vi "Target Defender Out.vi"(6 "Target Fora in":bool=TRUE, 8 "Field Size in":T1, 9 "Defensores":u32[](array[numeric]), 10 "total":i32, 11 "Ball":dbl[](array[numeric])) -> (2 "Target Fora out":bool=TRUE)   [LabVIEW 2016]
uses:
  Core/Field Size.ctl
panel:
  in  "Campo/2":dbl
  out "Posição dos Defensores":dbl[][](array[numeric])
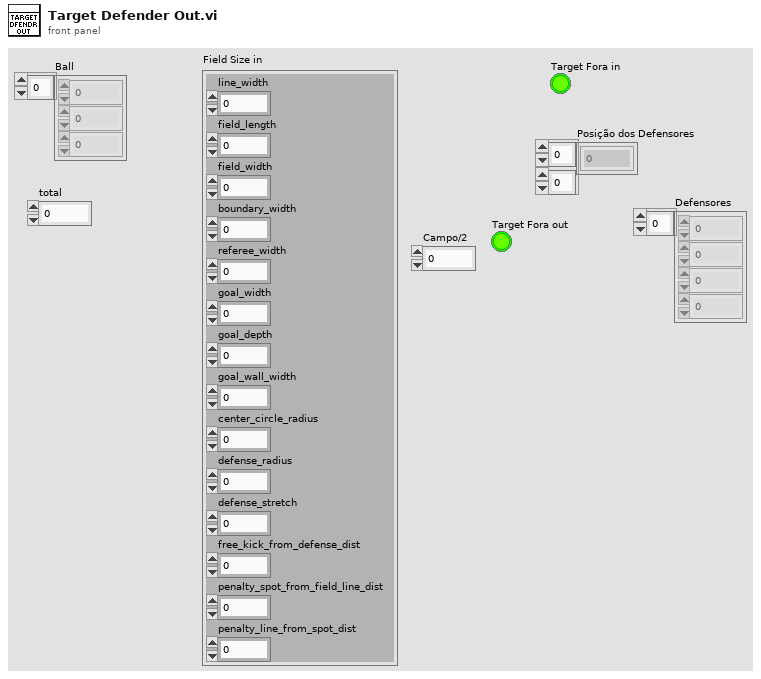
[diagram p1: front panel]
types:
  T1 = typedef "Field Size.ctl" = cluster{"line_width":u32, "field_length":u32, "field_width":u32, "boundary_width":u32, "referee_width":u32, "goal_width":u32, "goal_depth":u32, "goal_wall_width":u32, "center_circle_radius":u32, "defense_radius":u32, "defense_stretch":u32, "free_kick_from_defense_dist":u32, "penalty_spot_from_field_line_dist":u32, "penalty_line_from_spot_dist":u32}
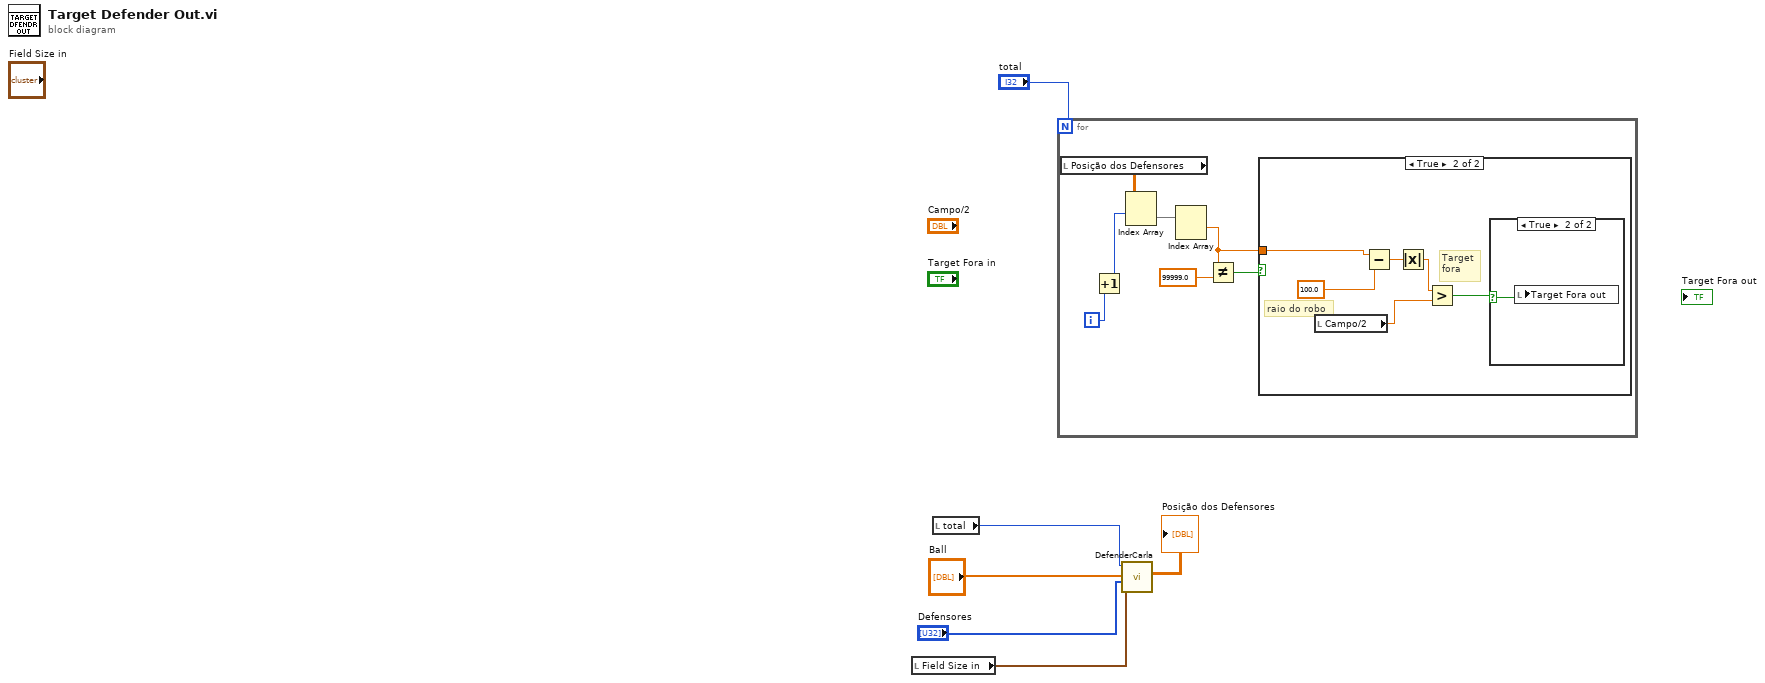
[diagram p0: block diagram]
diagram:
  n1 = local read "Field Size in"() -> (w5:T1)
  n2 = local read "total"() -> (w6:i32)
  n3 = for {
    N: "total" -> [_]
    i -> [w8]
    n4 = local read "Posição dos Defensores"() -> (w13:dbl[][])
    n5 = Increment(x=w8) -> (x+1=w7:i32)
    n6 = Index Array(array=w13, index (row)=w7) -> (element=w12:dbl[])  [unwired: 1 in]
    n7 = Index Array(array=w12) -> (element #1=w9:dbl)  [unwired: 2 in, 1 out]
    n8 = Not Equal?(x=w9, y=99999.0) -> (x != y?=w10:bool)
    n9 = case shown="True" w10 {
      tunnel: w9 -> [_ w14]
      frame False {
      }
      frame True {
        # "Target \nfora"
        # "raio do robo"
        n10 = local read "Campo/2"() -> (w16:dbl)
        n11 = Subtract(x=w14, y=100.0) -> (x-y=w18:dbl)
        n12 = Absolute Value(x=w18) -> (abs(x)=w17:dbl)
        n13 = Greater?(x=w17, y=w16) -> (0:w15:bool)
        n14 = case shown="True" w15 {
          selector: w15 -> [_ w20]
          frame False {
          }
          frame True {
            n15 = local write "Target Fora out"(w20) -> ()
          }
        }
      }
    }
  }
  n16 = call "DefenderCarla.vi"("Field Size in"=w5, "Defensores"="Defensores", "Ball"="Ball", "total"=w6) -> ("Posição dos Defensores"=→"Posição dos Defensores":dbl[][])  [unwired: 6 in]
